vi "Process.vi"(8 "error in":errorcluster, 11 "JKI.Robot.SMO":refnum<class "JKI.Robot.SMO.lvclass">) -> (0 "error out":errorcluster, 3 "JKI.Robot.SMO out":refnum<class "JKI.Robot.SMO.lvclass">)   [LabVIEW 2015, in "JKI.Robot.SMO.lvclass"]
doc: "---------------------------------------------------------------\nJKI State Machine Objects™\nhttp://jki.net/state-machine-objects/\nCopyright (C) 2005-2015, JKI <info@jki.net>\nALL RIGHTS RESERVEDJKI State Machine Objects (SMO) 1.0.0.5\nJKI - JKI\nCopyright (c) 2016, JKI"
uses:
  JKI.Robot.SMO.lvclass
  <vilib>/JKI/JKI SMO/SMO/Typedefs/Parent Call--Enum.ctl
  JKI.Robot.SMO.Base/JKI.Robot.SMO.Base.lvclass
  <vilib>/JKI/JKI SMO/SMO/SMO.lvclass
panel:
  out "Picture Out":picture
  # "JKI Robot (LabVIEW)"
  # "For instructions on how to use the JKI State Machine Objects, examples and video tutorials, visit:\nhttp://jki.net/state-machine-objects/\n\nJKI State Machine Objects™\nhttp://jki.net/state-machine-objects/\nCopyright (C) 2005-2015, JKI <info@jki.net>\nALL RIGHTS RESERVED"
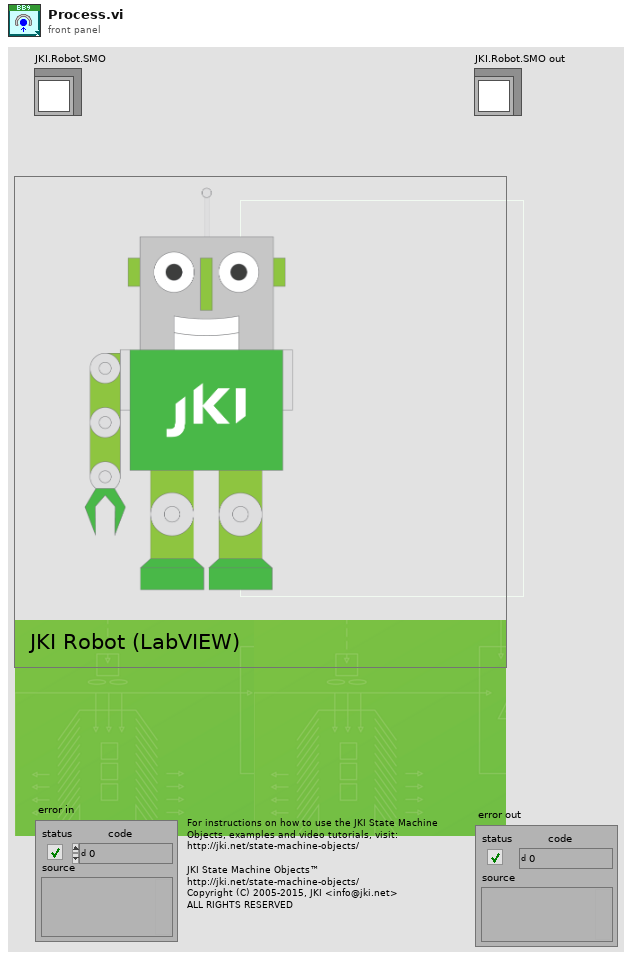
[diagram p1: front panel]
types:
  T1 = typedef "SMO.lvclass/Parent Call--Enum.ctl" = enum16{"Allows parent to run", "Does not request parent to run"}
  T2 = enum32{"invalid app kind", "Development System", "Run Time System", "Student Edition", "Embedded LabVIEW", "Evaluation", "Custom"}
  T3 = enum32{"Invalid", "Standard", "Closed", "Hidden", "Minimized", "Maximized"}
  T4 = typedef "JKI.Robot.SMO.lvclass/PrivateEvents--JKI.Robot.SMO.SetGrabberPosition.ctl" = dbl
  T5 = typedef "JKI.Robot.SMO.lvclass/PrivateEvents--Cluster.ctl" = cluster{"SetGrabberPosition":refnum<user-event>, "SetJointRotation":refnum<user-event>}
  T6 = typedef "JointType--Enum.ctl" = enum16{"A_Shoulder", "B_Elbow", "C_Wrist", "D_Base"}
  T7 = cluster{"Core":cluster{"Current VI Reference":refnum<vi>, "Close Panel on Exit?":bool, "error":errorcluster}, "Self Reference":refnum<class "JKI.Robot.SMO.lvclass">, "Your string data":string}
  T8 = cluster{"Current VI Reference":refnum<vi>, "Close Panel on Exit?":bool, "error":errorcluster}
  T9 = typedef "SMO.lvclass/Protected Events.ctl" = cluster{"StopProcesses":refnum<user-event>, "AbortProcesses":refnum<user-event>, "Config Changed":refnum<user-event>}
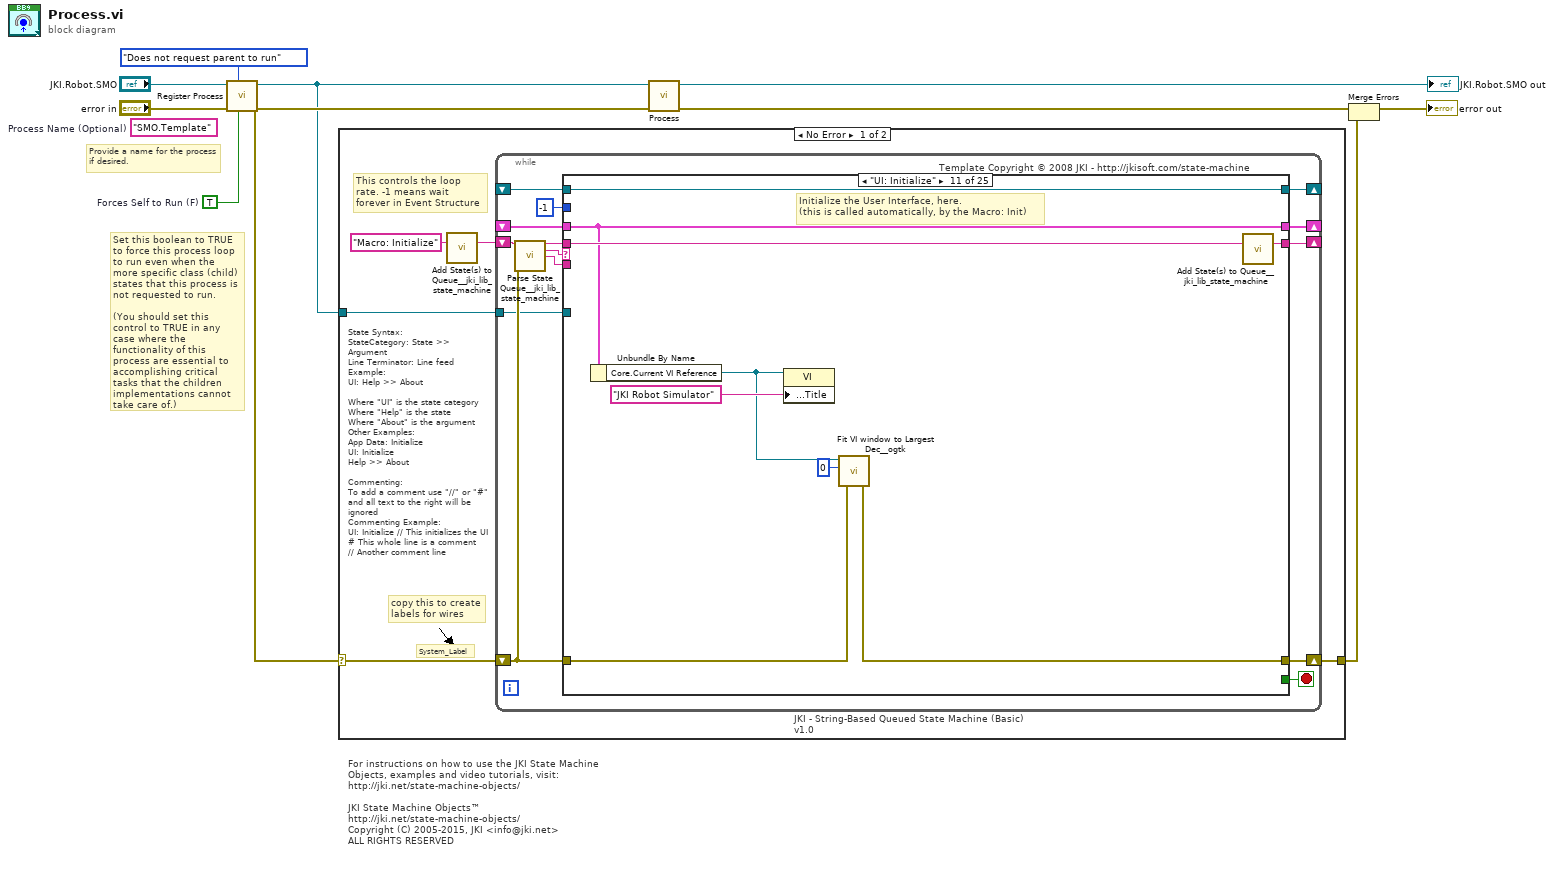
[diagram p0: block diagram]
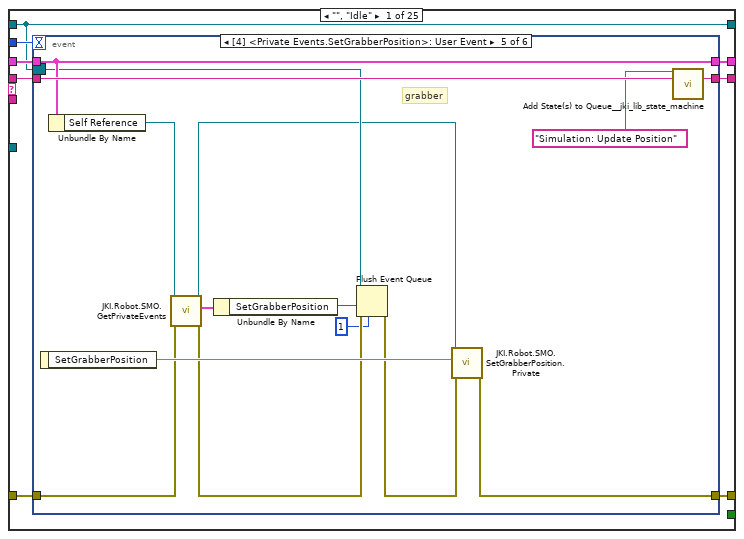
[diagram p2: hidden frame]
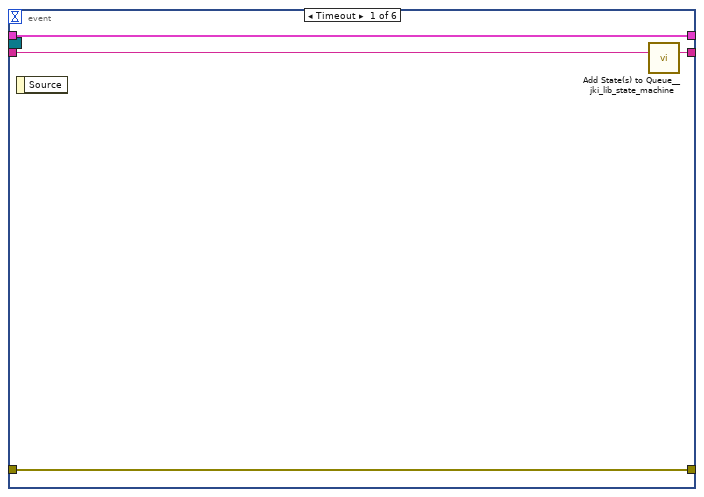
[diagram p3: hidden frame]
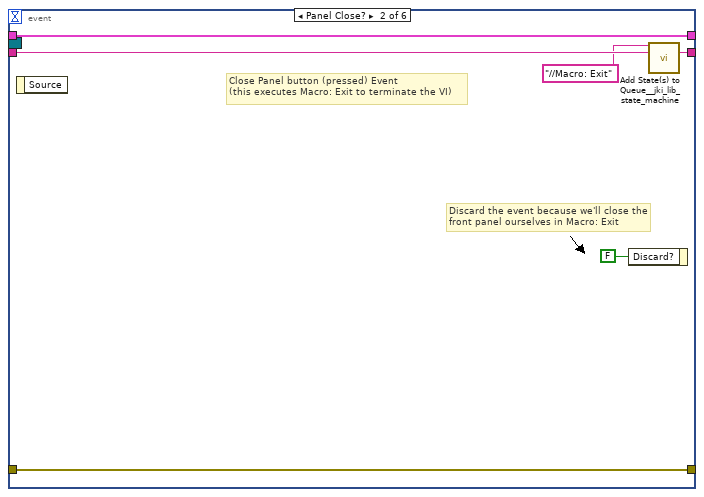
[diagram p4: hidden frame]
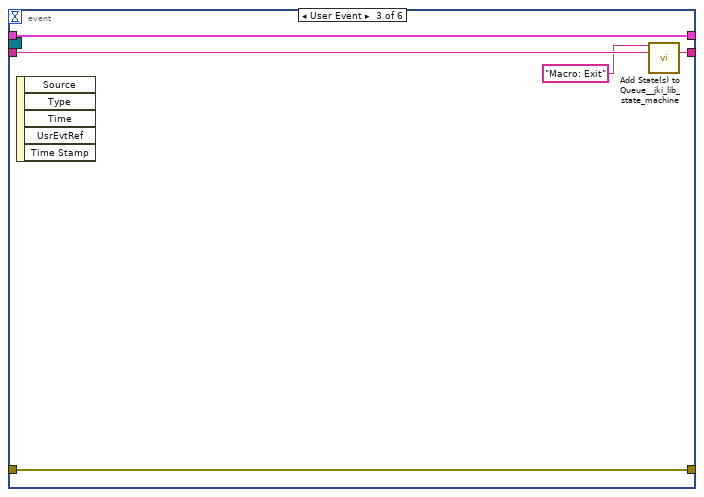
[diagram p5: hidden frame]
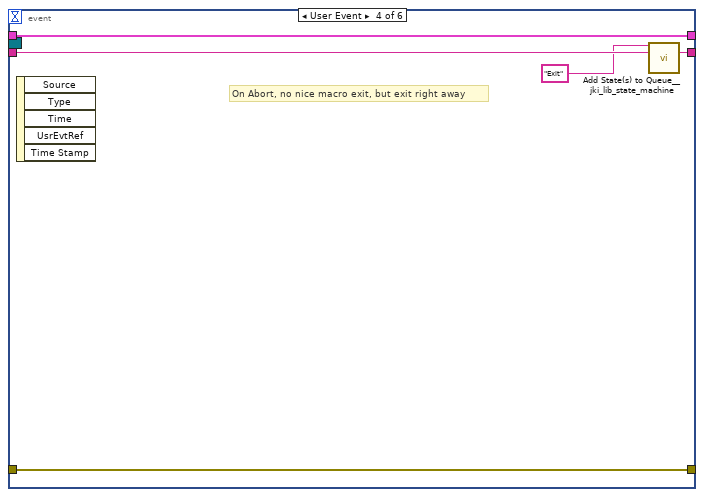
[diagram p6: hidden frame]
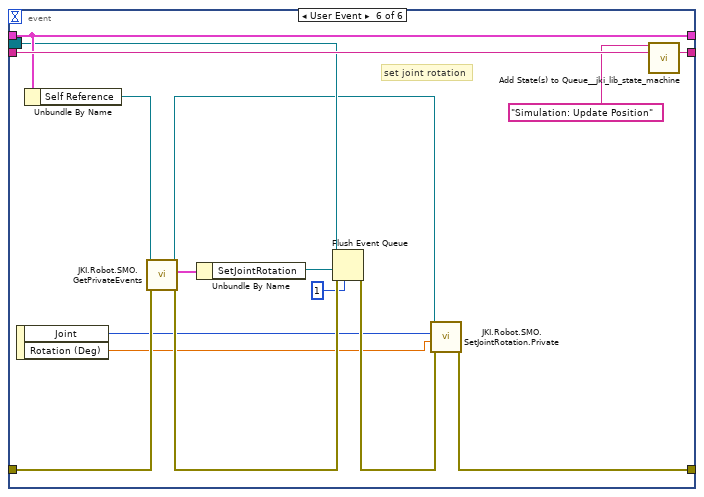
[diagram p7: hidden frame]
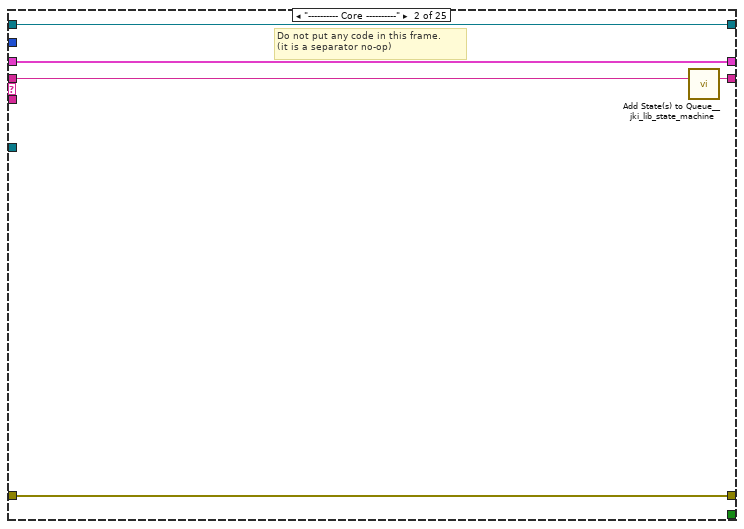
[diagram p8: hidden frame]
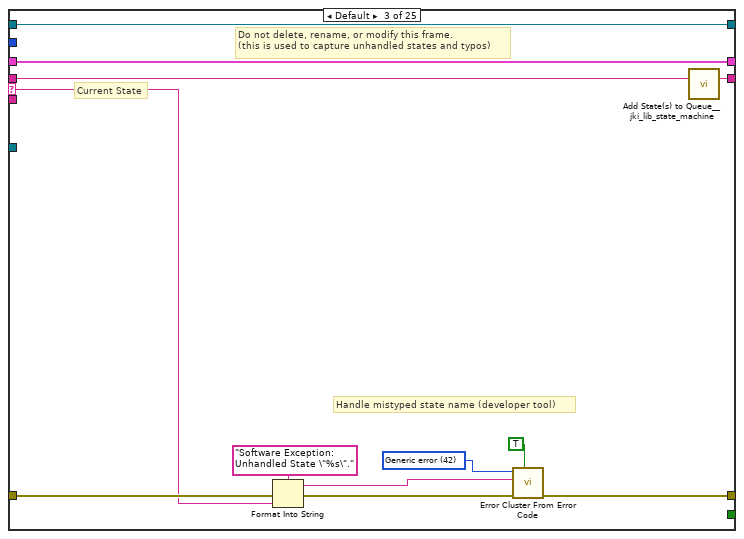
[diagram p9: hidden frame]
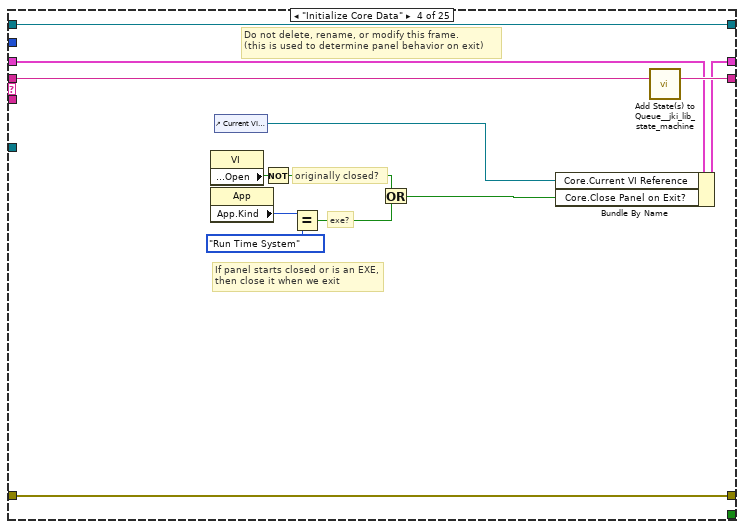
[diagram p10: hidden frame]
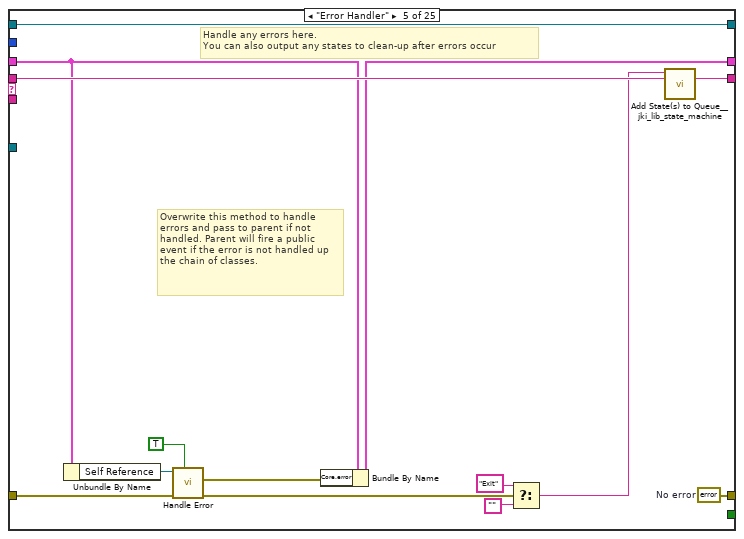
[diagram p11: hidden frame]
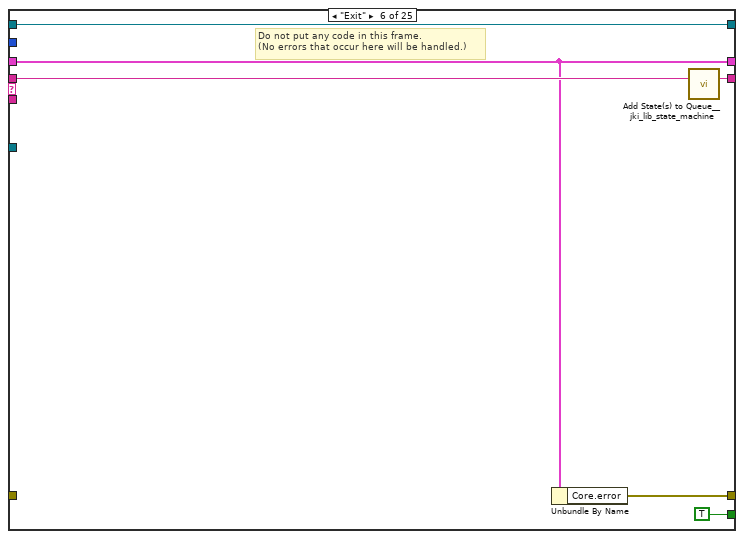
[diagram p12: hidden frame]
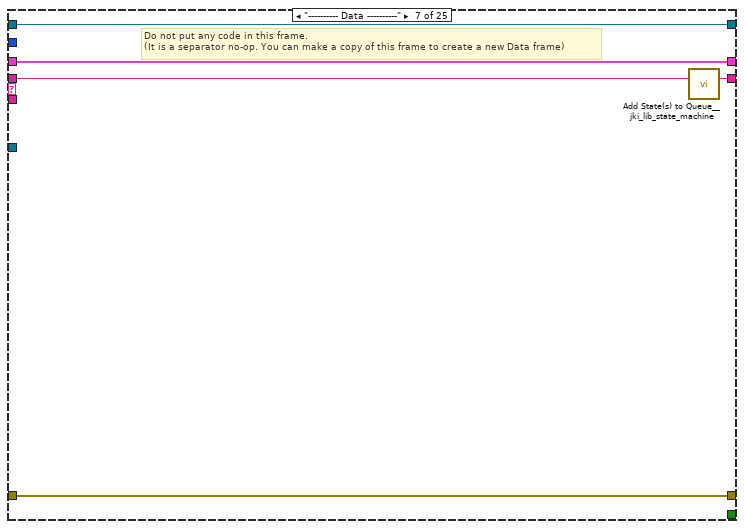
[diagram p13: hidden frame]
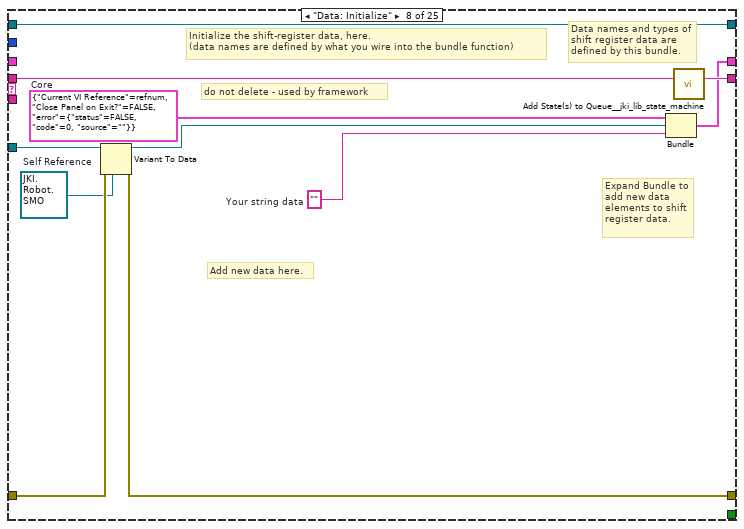
[diagram p14: hidden frame]
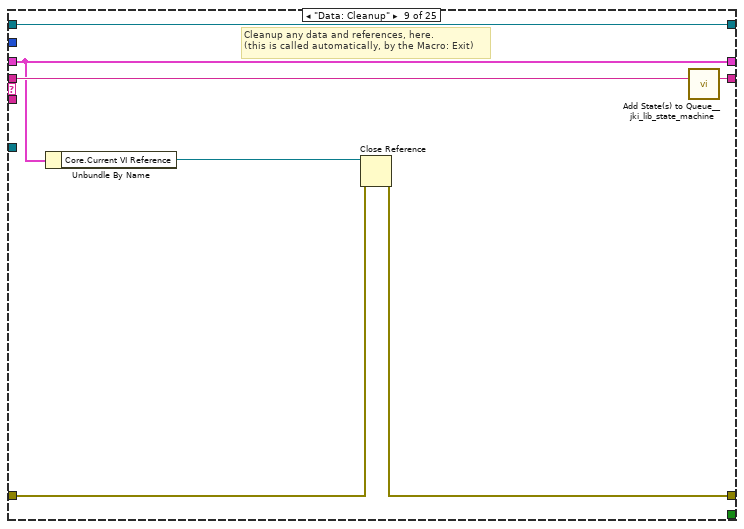
[diagram p15: hidden frame]
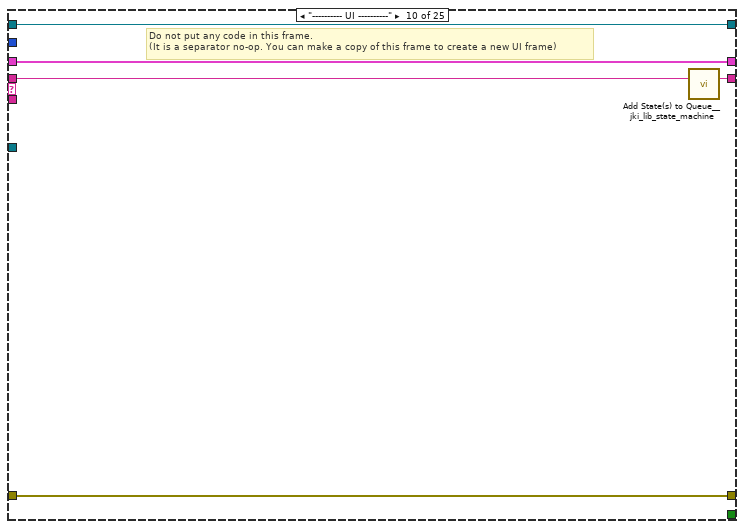
[diagram p16: hidden frame]
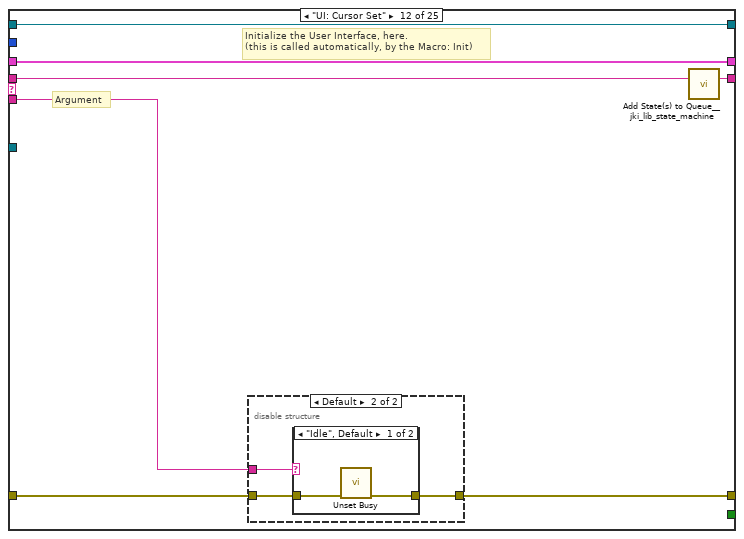
[diagram p17: hidden frame]
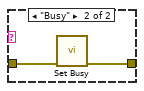
[diagram p19: hidden frame]
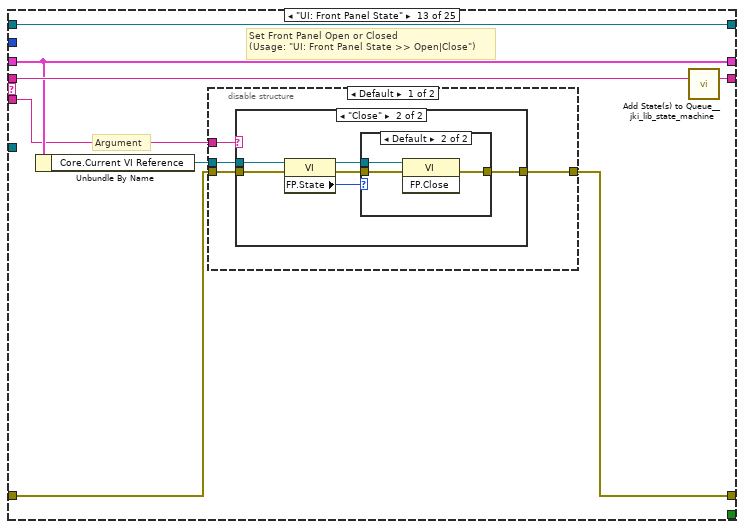
[diagram p20: hidden frame]
diagram:
  w1 = TRUE  # Forces Self to Run (F)
  (unwired) "SMO.Template"  # Process Name (Optional)
  # "Provide a name for the process\nif desired."
  # "Set this boolean to TRUE to force this process loop to run even when the more specific class (child) states that this process is not requested to run.\n\n(You should set this control to TRUE in any case where the functionality of this process are essential to accomplishing critical tasks that the children implementations cannot take care of.)"
  # "For instructions on how to use the JKI State Machine Objects, examples and video tutorials, visit:\nhttp://jki.net/state-machine-objects/\n\nJKI State Machine Objects™\nhttp://jki.net/state-machine-objects/\nCopyright (C) 2005-2015, JKI <info@jki.net>\nALL RIGHTS RESERVED"
  n1 = call <vilib>:"Register Process.vi"("Forces Self to Run (F)"=w1, "Parent Call"=Parent_Call--Enum."Does not request parent to run", "error in (no error)"="error in", "SMO"="JKI.Robot.SMO") -> ("error out"=w7:errorcluster, "SMO out"=w6:refnum<class "JKI.Robot.SMO.lvclass">)  [unwired: 6 in]
  n2 = case shown="No Error" w7 {
    selector: w7 -> [w12 w328]
    tunnel: w6 -> [w13 _]
    tunnel: [w11 w328] -> w3
    frame No Error {
      # "State Syntax:\nStateCategory: State >> Argument\nLine Terminator: Line feed\nExample:\nUI: Help >> About\n\nWhere \"UI\" is the state category\nWhere \"Help\" is the state\nWhere \"About\" is the argument\nOther Examples:\nApp Data: Initialize\nUI: Initialize\nHelp >> About\n\nCommenting:\nTo add a comment use \"//\" or \"#\" and all text to the right will be ignored\nCommenting Example:\nUI: Initialize // This initializes the UI\n# This whole line is a comment\n// Another comment line"
      # "copy this to create labels for wires"
      # "This controls the loop rate. -1 means wait forever in Event Structure"
      # "System_Label"
      n3 = call <vilib>:"Add State(s) to Queue__jki_lib_state_machine.vi"("State(s) in (\"\")"="Macro: Initialize") -> ("States Out"=w15:string)  [unwired: 14 in]
      n4 = while "JKI - String-Based Queued State Machine (Basic) v1.0" {
        shift-right: [w22] -> _
        shift-left: _ -> [w21]
        shift-right: [w25] -> w11
        shift-left: w12 -> [w19]
        shift-right: [w24] -> _
        shift-left: w15 -> [w26]
        tunnel: w13 -> [w18]
        shift-right: [w17] -> _
        shift-left: _ -> [w16]
        stop <- w23 stop-if-true
        # "Template Copyright © 2008 JKI - http://jkisoft.com/state-machine"
        n5 = call <vilib>:"Parse State Queue__jki_lib_state_machine.vi"("State Queue"=w26, "Error In (no error)"=w19) -> ("Remaining States"=w28:string, "Current State"=w29:string, "Arguments"=w27:string)  [unwired: 11 in]
        n6 = case shown="\"UI: Initialize\"" w29 {
          selector: w29 -> [_ _ w95 _ _ _ _ _ _ _ _ _ _ _ _ _ _ _ _ _ _ _ _ _ _]
          tunnel: w28 -> [w37 w93 w99 w118 w132 w138 w143 w154 w161 w166 w175 w182 w198 w230 w239 w253 w258 w269 w274 w287 w304 w309 w314 w319 w327]
          tunnel: w27 -> [_ _ _ _ _ _ _ _ _ _ _ w176 w192 _ _ _ _ _ _ _ _ _ _ _ _]
          tunnel: w21 -> [w35 w90 w97 w109 w121 w134 w140 _ w156 w163 w172 w180 w194 w227 w235 w244 w255 w266 w271 w285 w302 w307 w311 w317 w324]
          tunnel: [w34 w91 w101 w115 w123 w133 w141 w149 w157 w164 w168 w177 w195 w228 w237 w251 w256 w260 w272 w283 w300 w305 w310 w315 w322] -> w25
          tunnel: w19 -> [w33 w91 w100 w115 w128 _ w141 w150 w158 w164 w169 w178 w196 w228 w237 w251 w256 w261 w272 w284 w300 w305 w310 w315 w323]
          tunnel: [w36 w92 w98 w117 w131 w137 w142 w153 w160 w165 w174 w181 w197 w229 w238 w252 w257 w268 w273 w286 w303 w308 w313 w318 w326] -> w24
          tunnel: [_ _ _ _ _ TRUE _ _ _ _ _ _ _ _ _ _ _ _ _ _ _ _ _ _ _] -> w23
          tunnel: [w32 w90 w97 w116 w120 w134 w140 w152 w156 w163 w172 w180 w194 w227 w235 w244 w255 w266 w271 w285 w302 w307 w311 w317 w324] -> w22
          tunnel: -1 ("Timeout") -> [w31 _ _ _ _ _ _ _ _ _ _ _ _ _ _ _ _ _ _ _ _ _ _ _ _]
          tunnel: w18 -> [_ _ _ _ _ _ _ w147 _ _ _ _ _ _ _ _ _ _ _ _ _ _ _ _ _]
          tunnel: [w30 w89 w94 w106 w130 w135 w139 w145 w155 w162 w173 w179 w191 w226 w236 w245 w254 w267 w270 w275 w301 w306 w312 w316 w325] -> w17
          tunnel: w16 -> [w30 w89 w94 w106 w130 w135 w139 w145 w155 w162 w173 w179 w191 w226 w236 w245 w254 w267 w270 w279 w301 w306 w312 w316 w325]
          frame "", "Idle" {
            n7 = event shown="[4] <Private Events.SetGrabberPosition>: User Event" {
              selector: w30 -> [_ _ _ _ w65 w84]
              dyn-events: _ -> [_ _ _ _ _ _]
              timeout: w31 -> [_ _ _ _ _ _]
              tunnel: w37 -> [w41 w47 w52 w57 w72 w88]
              tunnel: [w40 w46 w51 w56 w71 w87] -> w36
              tunnel: w35 -> [w38 w44 w49 w54 w69 w85]
              tunnel: [w39 w45 w50 w55 w67 w76] -> w34
              tunnel: w33 -> [w39 w45 w50 w55 w60 w80]
              tunnel: [w38 w44 w49 w54 w69 w85] -> w32
              event Timeout {
                n8 = event-data() -> ()  [unwired: 1 in, 1 out]
                n9 = call <vilib>:"Add State(s) to Queue__jki_lib_state_machine.vi"("State(s) in (\"\")"=w41) -> ("States Out"=w40:string)  [unwired: 14 in]
              }
              event Panel Close? {
                # "Discard the event because we'll close the front panel ourselves in Macro: Exit"
                # "Close Panel button (pressed) Event\n(this executes Macro: Exit to terminate the VI)"
                n10 = event-data() -> ()  [unwired: 1 in, 1 out]
                n11 = event-data("Discard?"=FALSE) -> ()  [unwired: 1 in, 1 out]
                n12 = call <vilib>:"Add State(s) to Queue__jki_lib_state_machine.vi"("State(s) in Front (\"\")"="//Macro: Exit", "State(s) in (\"\")"=w47) -> ("States Out"=w46:string)  [unwired: 13 in]
              }
              event User Event {
                n13 = event-data() -> ()  [unwired: 1 in, 5 out]
                n14 = call <vilib>:"Add State(s) to Queue__jki_lib_state_machine.vi"("State(s) in Front (\"\")"="Macro: Exit", "State(s) in (\"\")"=w52) -> ("States Out"=w51:string)  [unwired: 13 in]
              }
              event User Event {
                # "On Abort, no nice macro exit, but exit right away"
                n15 = event-data() -> ()  [unwired: 1 in, 5 out]
                n16 = call <vilib>:"Add State(s) to Queue__jki_lib_state_machine.vi"("State(s) in Front (\"\")"="Exit", "State(s) in (\"\")"=w57) -> ("States Out"=w56:string)  [unwired: 13 in]
              }
              event User Event {
                # "grabber"
                n17 = event-data() -> ("SetGrabberPosition"=w68:T4)  [unwired: 1 in]
                n18 = Unbundle By Name(w69) -> ("Self Reference"=w62:refnum<class "JKI.Robot.SMO.lvclass">)
                n19 = call "JKI.Robot.SMO.GetPrivateEvents.vi"("error in (no error)"=w60, "JKI.Robot.SMO"=w62) -> ("error out"=w59:errorcluster, "Private Events"=w64:T5, "JKI.Robot.SMO out"=w61:refnum<class "JKI.Robot.SMO.lvclass">)  [unwired: 7 in]
                n20 = Unbundle By Name(w64) -> ("SetGrabberPosition"=w63:refnum<user-event>)
                n21 = Flush Event Queue(0:w65, 2:w63, 3:w59, 5:1 ("keep most recent")) -> (11:w66:errorcluster)  [unwired: 2 in, 2 out]
                n22 = call "JKI.Robot.SMO.SetGrabberPosition.Private.vi"("error in (no error)"=w66, "Robot Position.Claw Value"=w68, "JKI.Robot.SMO"=w61) -> ("error out"=w67:errorcluster)  [unwired: 7 in, 1 out]
                n23 = call <vilib>:"Add State(s) to Queue__jki_lib_state_machine.vi"("State(s) in Front (\"\")"="Simulation: Update Position", "State(s) in (\"\")"=w72) -> ("States Out"=w71:string)  [unwired: 13 in]
              }
              event User Event {
                # "set joint rotation"
                n24 = event-data() -> ("Joint"=w75:T6, "Rotation (Deg)"=w74:dbl)  [unwired: 1 in]
                n25 = Unbundle By Name(w85) -> ("Self Reference"=w81:refnum<class "JKI.Robot.SMO.lvclass">)
                n26 = call "JKI.Robot.SMO.GetPrivateEvents.vi"("error in (no error)"=w80, "JKI.Robot.SMO"=w81) -> ("error out"=w79:errorcluster, "Private Events"=w83:T5, "JKI.Robot.SMO out"=w78:refnum<class "JKI.Robot.SMO.lvclass">)  [unwired: 7 in]
                n27 = Unbundle By Name(w83) -> ("SetJointRotation"=w82:refnum<user-event>)
                n28 = Flush Event Queue(0:w84, 2:w82, 3:w79, 5:1 ("keep most recent")) -> (11:w77:errorcluster)  [unwired: 2 in, 2 out]
                n29 = call "JKI.Robot.SMO.SetJointRotation.Private.vi"("error in (no error)"=w77, "Robot Position.Claw Value"=w74, "Joint"=w75, "JKI.Robot.SMO"=w78) -> ("error out"=w76:errorcluster)  [unwired: 6 in, 1 out]
                n30 = call <vilib>:"Add State(s) to Queue__jki_lib_state_machine.vi"("State(s) in Front (\"\")"="Simulation: Update Position", "State(s) in (\"\")"=w88) -> ("States Out"=w87:string)  [unwired: 13 in]
              }
            }
          }
          frame "---------- Core ----------" {
            # "Do not put any code in this frame.\n(it is a separator no-op)"
            n31 = call <vilib>:"Add State(s) to Queue__jki_lib_state_machine.vi"("State(s) in (\"\")"=w93) -> ("States Out"=w92:string)  [unwired: 14 in]
          }
          frame Default {
            w104 = 42 items=["No error", "Argument error", "Memory is full", "Out of zone", "End of file", "File already open", "Generic file I/O error", "File not found", "File permission error", "Disk is full", "Duplicate path", "Too many files open", "System feature not enabled", "Resource file not found", "Cannot add resource", "Resource not found", "Image not found", "Image memory error", "Pen does not exist", "Config type invalid", "Config token not found", "Config parse error", "Config memory error", "Bad external code format", "Bad external code offset", "External code not present", "Null window", "Destroy window error", "Null menu", "Print aborted", "Bad print record", "Print driver error", "Windows error during printing", "Memory error during printing", "Print dialog error", "Generic print error", "Invalid device refnum", "Device not found", "Device parameter error", "Device unit error", "Cannot open device", "Device call aborted", "Generic error", "Cancelled by user", "Object ID too low", "Object ID too high", "Object not in heap", "Unknown heap", "Unknown object (invalid DefProc)", "Unknown object (DefProc not in table)", "Message out of range", "Invalid (null) method", "Unknown message", "Manager call not supported", "Bad address", "Network operation in progress", "Network operation timed out", "Connection is busy", "Network attribute not supported", "Network error", "Address in use", "System out of memory", "Connection aborted", "Connection refused", "Not connected", "Already connected", "Connection closed", "Initialization error (interapplication manager)", "Bad occurrence", "Wait on unbound occurrence handler", "Occurrence queue overflow", "Datalog type conflict", "Unused", "Unrecognized type (interapplication manager)", "Memory corrupt", "Failed to make temporary DLL", "Old CIN version", "Drag socket not found", "Failed to load drop-object", "Failed to register OLE object", "Failed to release OLE object", "Format specifier type mismatch", "Unknown format specifier", "Too few format specifiers", "Too many format specifiers", "Scan failed", "Newer CIN version", "Error converting to variant", "Runtime menu error", "Password tampered", "Variant attribute not found", "Incompatible variant data type", "Event data is not available", "Event Store is not present", "Occurrence is not found", "Event Queue is not created", "Event info is not available", "Refnum passed is NULL", "Error retrieving Class GUID", "Error retrieving CoClass GUID", "Error retrieving TypeLib GUID.", "Bad built application magic bytes.", "Specific driver is different from the specific driver associated with the Logical Name.", "There is no session opened to the class driver.", "Max Error", "MAX - Error with config objects", "MAX - Error loading configuration", "MAX - Group not supported"]
            # "Current State"
            # "Do not delete, rename, or modify this frame.\n(this is used to capture unhandled states and typos)"
            # "Handle mistyped state name (developer tool)"
            n32 = Format Into String(format string="Software Exception: Unhandled State \"%s\"." ("message"), error in=w100, w95) -> (resulting string=w103:string, error out=w102:errorcluster)  [unwired: 1 in]
            n33 = call <vilib>:"Error Cluster From Error Code.vi"("show call chain? (False)"=TRUE, "error in (no error)"=w102, "error message (\"\")"=w103, "error code (0)"=w104) -> ("error out"=w101:errorcluster)  [unwired: 5 in]
            n34 = call <vilib>:"Add State(s) to Queue__jki_lib_state_machine.vi"("State(s) in (\"\")"=w99) -> ("States Out"=w98:string)  [unwired: 14 in]
          }
          frame "Initialize Core Data" {
            # "Do not delete, rename, or modify this frame.\n(this is used to determine panel behavior on exit)"
            # "originally closed?"
            # "exe?"
            # "If panel starts closed or is an EXE, then close it when we exit"
            n35 = property class="VI"() -> ("Front Panel.Open"=w114:bool)  [unwired: 2 in, 2 out]
            n36 = property class="App"() -> ("App.Kind"=w113:T2)  [unwired: 2 in, 2 out]
            n37 = control-ref of="Current VI Reference"() -> (w107:refnum<vi>)
            n38 = Not(x=w114) -> (.not. x?=w111:bool)
            n39 = Equal?(x=w113, y=T2."Run Time System" ("Application:Kind")) -> (x = y?=w110:bool)
            n40 = Or(x=w111, y=w110) -> (x .or. y?=w108:bool)
            n41 = Bundle By Name(cluster=w109, "Core.Current VI Reference"=w107, "Core.Close Panel on Exit?"=w108) -> (w116:T7)
            n42 = call <vilib>:"Add State(s) to Queue__jki_lib_state_machine.vi"("State(s) in (\"\")"=w118) -> ("States Out"=w117:string)  [unwired: 14 in]
          }
          frame "Error Handler" {
            w123 = errorcluster {"status"=FALSE, "code"=0, "source"=""}  # No error
            # "Overwrite this method to handle errors and pass to parent if not handled. Parent will fire a public event if the error is not handled up the chain of classes."
            # "Handle any errors here.\nYou can also output any states to clean-up after errors occur"
            n43 = Unbundle By Name(w121) -> ("Self Reference"=w129:refnum<class "JKI.Robot.SMO.lvclass">)
            n44 = call-dynamic "Handle Error.vi"("Stop on Unhandled Error (T)"=TRUE, "error in"=w128, "SMO"=w129) -> ("handling error"=w124:errorcluster, "Unhandled error"=w122:errorcluster)  [unwired: 6 in, 1 out]
            n45 = Bundle By Name(cluster=w121, "Core.error"=w122) -> (w120:T7)
            n46 = Select(t="Exit", s=w124, f="") -> (s? t:f=w125:string)
            n47 = call <vilib>:"Add State(s) to Queue__jki_lib_state_machine.vi"("State(s) in Front (\"\")"=w125, "State(s) in (\"\")"=w132) -> ("States Out"=w131:string)  [unwired: 13 in]
          }
          frame "Exit" {
            # "Do not put any code in this frame.\n(No errors that occur here will be handled.)"
            n48 = Unbundle By Name(w134) -> ("Core.error"=w133:errorcluster)
            n49 = call <vilib>:"Add State(s) to Queue__jki_lib_state_machine.vi"("State(s) in (\"\")"=w138) -> ("States Out"=w137:string)  [unwired: 14 in]
          }
          frame "---------- Data ----------" {
            # "Do not put any code in this frame.\n(It is a separator no-op. You can make a copy of this frame to create a new Data frame)"
            n50 = call <vilib>:"Add State(s) to Queue__jki_lib_state_machine.vi"("State(s) in (\"\")"=w143) -> ("States Out"=w142:string)  [unwired: 14 in]
          }
          frame "Data: Initialize" {
            w144 = T8 {"Current VI Reference"=refnum, "Close Panel on Exit?"=FALSE, "error"={"status"=FALSE, "code"=0, "source"=""}}  # Core
            w148 = refnum<class "JKI.Robot.SMO.lvclass"> refnum  # Self Reference
            w151 = ""  # Your string data
            # "do not delete - used by framework"
            # "Expand Bundle to add new data elements to shift register data."
            # "Add new data here."
            # "Data names and types of shift register data are defined by this bundle."
            # "Initialize the shift-register data, here.\n(data names are defined by what you wire into the bundle function)"
            n51 = Variant To Data(error in=w150, type=w148, Variant=w147) -> (data=w146:refnum<class "JKI.Robot.SMO.lvclass">, error out=w149:errorcluster)
            n52 = Bundle("Core"=w144, "Self Reference"=w146, "Your string data"=w151) -> (w152:T7)  [unwired: 1 in]
            n53 = call <vilib>:"Add State(s) to Queue__jki_lib_state_machine.vi"("State(s) in (\"\")"=w154) -> ("States Out"=w153:string)  [unwired: 14 in]
          }
          frame "Data: Cleanup" {
            # "Cleanup any data and references, here.\n(this is called automatically, by the Macro: Exit)"
            n54 = Unbundle By Name(w156) -> ("Core.Current VI Reference"=w159:refnum<vi>)
            n55 = Close Reference(reference=w159, error in (no error)=w158) -> (error out=w157:errorcluster)
            n56 = call <vilib>:"Add State(s) to Queue__jki_lib_state_machine.vi"("State(s) in (\"\")"=w161) -> ("States Out"=w160:string)  [unwired: 14 in]
          }
          frame "---------- UI ----------" {
            # "Do not put any code in this frame.\n(It is a separator no-op. You can make a copy of this frame to create a new UI frame)"
            n57 = call <vilib>:"Add State(s) to Queue__jki_lib_state_machine.vi"("State(s) in (\"\")"=w166) -> ("States Out"=w165:string)  [unwired: 14 in]
          }
          frame "UI: Initialize" {
            # "Initialize the User Interface, here.\n(this is called automatically, by the Macro: Init)"
            n58 = Unbundle By Name(w172) -> ("Core.Current VI Reference"=w170:refnum<vi>)
            n59 = property class="VI"(reference=w170, "Front Panel.Title"="JKI Robot Simulator" ("Front Panel Window:Title")) -> ()  [unwired: 1 in, 2 out]
            n60 = call <userlib>:"Fit VI window to Largest Dec__ogtk.vi"("error in (no error)"=w169, "border spacing (2 px)"=0, "VI Ref (calling VI)"=w170) -> ("error out"=w168:errorcluster)  [unwired: 3 in, 1 out]
            n61 = call <vilib>:"Add State(s) to Queue__jki_lib_state_machine.vi"("State(s) in (\"\")"=w175) -> ("States Out"=w174:string)  [unwired: 14 in]
          }
          frame "UI: Cursor Set" {
            # "Argument"
            # "Initialize the User Interface, here.\n(this is called automatically, by the Macro: Init)"
            n62 = disable-structure shown="Default" {
              disable-tunnel: w178 -> [w183 w186]
              disable-tunnel: [w183 w185] -> w177
              disable-tunnel: w176 -> [_ w184]
              frame condition #0 {
              }
              frame condition #1 (active) {
                n63 = case shown="\"Idle\", Default" w184 {
                  tunnel: w186 -> [w188 w190]
                  tunnel: [w187 w189] -> w185
                  frame "Idle", Default {
                    n64 = call <vilib>:"Unset Busy.vi"("error in (no error)"=w188) -> ("error out"=w187:errorcluster)  [unwired: 10 in]
                  }
                  frame "Busy" {
                    n65 = call <vilib>:"Set Busy.vi"("error in (no error)"=w190) -> ("error out"=w189:errorcluster)  [unwired: 9 in, 1 out]
                  }
                }
              }
            }
            n66 = call <vilib>:"Add State(s) to Queue__jki_lib_state_machine.vi"("State(s) in (\"\")"=w182) -> ("States Out"=w181:string)  [unwired: 14 in]
          }
          frame "UI: Front Panel State" {
            # "Argument"
            # "Set Front Panel Open or Closed\n(Usage: \"UI: Front Panel State >> Open|Close\")"
            n67 = Unbundle By Name(w194) -> ("Core.Current VI Reference"=w193:refnum<vi>)
            n68 = disable-structure shown="Default" {
              disable-tunnel: w196 -> [w202 w225]
              disable-tunnel: [w201 w225] -> w195
              disable-tunnel: w193 -> [w200 _]
              disable-tunnel: w192 -> [w199 _]
              frame condition #0 (active) {
                n69 = case shown="\"Close\"" w199 {
                  tunnel: w202 -> [w206 w219]
                  tunnel: [w208 w220] -> w201
                  tunnel: w200 -> [w207 w217]
                  frame "Open", Default {
                    n70 = property class="VI"(reference=w207, error in=w206) -> (reference out=w204:refnum<vi>, error out=w205:errorcluster, "FP.State"=w203:T3)
                    n71 = case shown="\"Closed\"" w203 {
                      tunnel: [w211 w214] -> w208
                      tunnel: w205 -> [w210 w214]
                      tunnel: w204 -> [w209 _]
                      frame "Closed" {
                        n72 = invoke class="VI" method="FP.Open"(reference=w209, error in=w210, "Activate"=TRUE, "State"=T3."Standard") -> (error out=w211:errorcluster)  [unwired: 1 in, 4 out]
                      }
                      frame Default {
                      }
                    }
                  }
                  frame "Close" {
                    n73 = property class="VI"(reference=w217, error in=w219) -> (reference out=w216:refnum<vi>, error out=w218:errorcluster, "FP.State"=w215:T3)
                    n74 = case shown="Default" w215 {
                      tunnel: [w221 w224] -> w220
                      tunnel: w218 -> [w221 w223]
                      tunnel: w216 -> [_ w222]
                      frame "Invalid", "Closed" {
                      }
                      frame Default {
                        n75 = invoke class="VI" method="FP.Close"(reference=w222, error in=w223) -> (error out=w224:errorcluster)  [unwired: 1 in, 2 out]
                      }
                    }
                  }
                }
              }
              frame condition #1 {
              }
            }
            n76 = call <vilib>:"Add State(s) to Queue__jki_lib_state_machine.vi"("State(s) in (\"\")"=w198) -> ("States Out"=w197:string)  [unwired: 14 in]
          }
          frame "---------- Macro ----------" {
            # "Do not put any code in this frame.\n(It is a separator no-op. You can make a copy of this frame to create a new Macro frame)"
            n77 = call <vilib>:"Add State(s) to Queue__jki_lib_state_machine.vi"("State(s) in (\"\")"=w230) -> ("States Out"=w229:string)  [unwired: 14 in]
          }
          frame "Macro: Initialize" {
            w233 = "UI: Initialize\nSimulation: Update Position\nUI: Front Panel State >> Open"  # UI: Initialize Simulation: Update Position UI: Front Panel State >> Open
            # "Initialization Macro\n(This is called once, when the VI starts)"
            n78 = call <vilib>:"Add State(s) to Queue__jki_lib_state_machine.vi"("State(s) in Front (\"\")"="Data: Initialize\nInitialize Core Data\nEvents: Register", "State(s) in (\"\")"="Process: Sync", "State(s) at Back (\"\")"=w233) -> ("States Out"=w232:string)  [unwired: 12 in]
            n79 = call <vilib>:"Add State(s) to Queue__jki_lib_state_machine.vi"("State(s) in Front (\"\")"=w232, "State(s) in (\"\")"=w239) -> ("States Out"=w238:string)  [unwired: 13 in]
          }
          frame "Macro: Exit" {
            # "Exit Macro\n(This is called once, when the VI exits)"
            n80 = Unbundle By Name(w244) -> ("Core.Close Panel on Exit?"=w250:bool)
            n81 = Select(t="UI: Front Panel State >> Close", s=w250, f="") -> (s? t:f=w247:string)
            n82 = call <vilib>:"Add State(s) to Queue__jki_lib_state_machine.vi"("State(s) in Front (\"\")"="Data: Cleanup\nEvents: Unregister", "State(s) in (\"\")"="Process: Sync", "State(s) at Back (\"\")"="Exit") -> ("States Out"=w241:string)  [unwired: 12 in]
            n83 = call <vilib>:"Add State(s) to Queue__jki_lib_state_machine.vi"("State(s) in (\"\")"=w247, "State(s) at Back (\"\")"=w241) -> ("States Out"=w246:string)  [unwired: 13 in]
            n84 = call <vilib>:"Add State(s) to Queue__jki_lib_state_machine.vi"("State(s) in Front (\"\")"=w246, "State(s) in (\"\")"=w253) -> ("States Out"=w252:string)  [unwired: 13 in]
          }
          frame "---------- Process ----------" {
            # "Template Separator\n(You can make a copy of, or modify, this frame)"
            n85 = call <vilib>:"Add State(s) to Queue__jki_lib_state_machine.vi"("State(s) in (\"\")"=w258) -> ("States Out"=w257:string)  [unwired: 14 in]
          }
          frame "Process: Sync" {
            n86 = Unbundle By Name(w266) -> ("Self Reference"=w262:refnum<class "JKI.Robot.SMO.lvclass">)
            n87 = call <vilib>:"WaitOnProcessSync.vi"("error in (no error)"=w261, "SMO"=w262) -> ("error out"=w260:errorcluster, "Don't run?"=w265:bool)  [unwired: 7 in, 1 out]
            n88 = Select(t="Data: Cleanup\nEvents: Unregister\nExit", s=w265, f="") -> (s? t:f=w259:string)
            n89 = call <vilib>:"Add State(s) to Queue__jki_lib_state_machine.vi"("State(s) in Front (\"\")"=w259, "State(s) in (\"\")"=w269) -> ("States Out"=w268:string)  [unwired: 13 in]
          }
          frame "---------- Events ----------" {
            # "Template Separator\n(You can make a copy of, or modify, this frame)"
            n90 = call <vilib>:"Add State(s) to Queue__jki_lib_state_machine.vi"("State(s) in (\"\")"=w274) -> ("States Out"=w273:string)  [unwired: 14 in]
          }
          frame "Events: Register" {
            # "Self Events (API Calls)"
            # "Base Class Protected Events"
            n91 = Unbundle By Name(w285) -> ("Self Reference"=w281:refnum<class "JKI.Robot.SMO.lvclass">)
            n92 = call <vilib>:"GetProtectedEvents.vi"("error in (no error)"=w284, "SMO"=w281) -> ("error out"=w277:errorcluster, "SMO Protected Events"=w282:T9, "SMO out"=w278:refnum<class "JKI.Robot.SMO.lvclass">)  [unwired: 7 in]
            n93 = call "JKI.Robot.SMO.GetPrivateEvents.vi"("error in (no error)"=w277, "JKI.Robot.SMO"=w278) -> ("Private Events"=w276:T5)  [unwired: 7 in, 2 out]
            n94 = Not A Number/Path/Refnum?(number/path/refnum=w279) -> (NaN/Path/Refnum?=w280:bool)
            n95 = case shown="True" w280 {
              tunnel: [w292 w298] -> w283
              tunnel: [w288 w297] -> w275
              tunnel: w282 -> [w291 w296]
              tunnel: w277 -> [w290 w295]
              tunnel: w279 -> [_ w294]
              tunnel: w276 -> [w289 w293]
              frame True {
                # "Expand to add\nmore events"
                n96 = register-events(error in=w290, w291, w289) -> (reference out=w288:refnum<event-registration>, error out=w292:errorcluster)  [unwired: 1 in]
              }
              frame False {
                n97 = register-events(reference=w294, error in=w295, w296, w293) -> (reference out=w297:refnum<event-registration>, error out=w298:errorcluster)
              }
            }
            n98 = call <vilib>:"Add State(s) to Queue__jki_lib_state_machine.vi"("State(s) in (\"\")"=w287) -> ("States Out"=w286:string)  [unwired: 14 in]
          }
          frame "Events: Unregister" {
            n99 = Unregister For Events(event registration refnum=w301, error in=w300) -> (error out=w299:errorcluster)
            n100 = call <vilib>:"Clear Errors.vi"("error in (no error)"=w299) -> ()  [unwired: 5 in, 2 out]
            n101 = call <vilib>:"Add State(s) to Queue__jki_lib_state_machine.vi"("State(s) in (\"\")"=w304) -> ("States Out"=w303:string)  [unwired: 14 in]
          }
          frame "---------- API ----------" {
            n102 = call <vilib>:"Add State(s) to Queue__jki_lib_state_machine.vi"("State(s) in (\"\")"=w309) -> ("States Out"=w308:string)  [unwired: 14 in]
          }
          frame "API: NewData" {
            n103 = call <vilib>:"Add State(s) to Queue__jki_lib_state_machine.vi"("State(s) in (\"\")"=w314) -> ("States Out"=w313:string)  [unwired: 14 in]
          }
          frame "---------Simulation-----------" {
            n104 = call <vilib>:"Add State(s) to Queue__jki_lib_state_machine.vi"("State(s) in (\"\")"=w319) -> ("States Out"=w318:string)  [unwired: 14 in]
          }
          frame "Simulation: Update Position" {
            n105 = Unbundle By Name(w324) -> ("Self Reference"=w321:refnum<class "JKI.Robot.SMO.lvclass">)
            n106 = call "JKI.Robot.DrawRobot.vi"("error in (no error)"=w323, "JKI.Robot.SMO"=w321) -> ("error out"=w322:errorcluster, "Picture Out"=→"Picture Out":picture)  [unwired: 7 in, 1 out]
            n107 = call <vilib>:"Add State(s) to Queue__jki_lib_state_machine.vi"("State(s) in (\"\")"=w327) -> ("States Out"=w326:string)  [unwired: 14 in]
          }
        }
      }
    }
    frame Error {
    }
  }
  n108 = call-parent "Process.vi"("error in"=w7, "JKI.Robot.SMO.Base"=w6) -> ("error out"=w4:errorcluster, "JKI.Robot.SMO.Base out"=→"JKI.Robot.SMO out":refnum<class "JKI.Robot.SMO.lvclass">)  [unwired: 8 in]
  n109 = Merge Errors(w4, w3) -> (→"error out":errorcluster)
